vi "Arm Mode.vi"() -> ()   [LabVIEW 2015]
uses:
  Global Angle.vi
  Global Distance.vi
panel:
  in  "last 2":dbl
  in  "last":dbl
  out "delta1":dbl
  out "delta2":dbl
  out "delta3":dbl
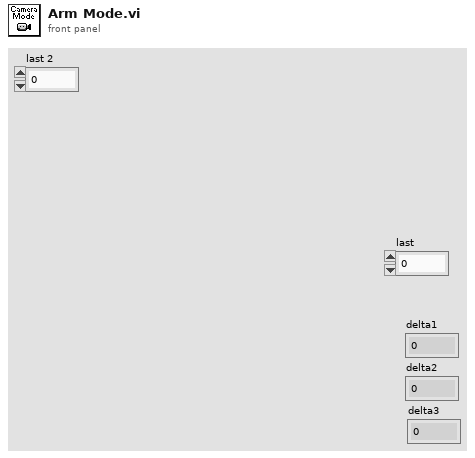
[diagram p1: front panel]
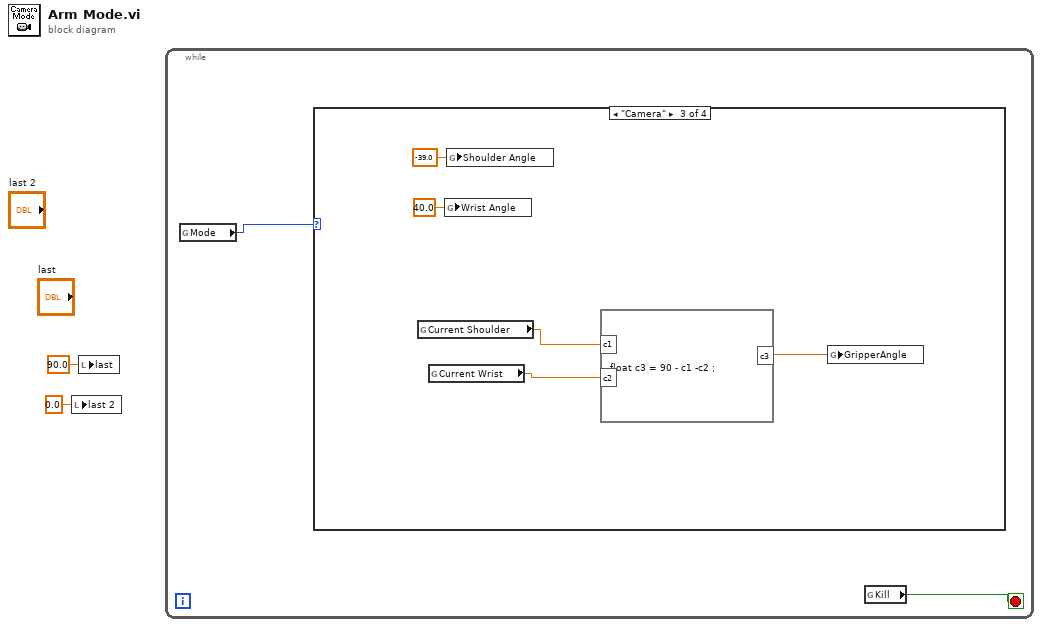
[diagram p0: block diagram]
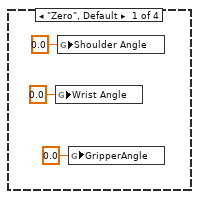
[diagram p2: hidden frame]
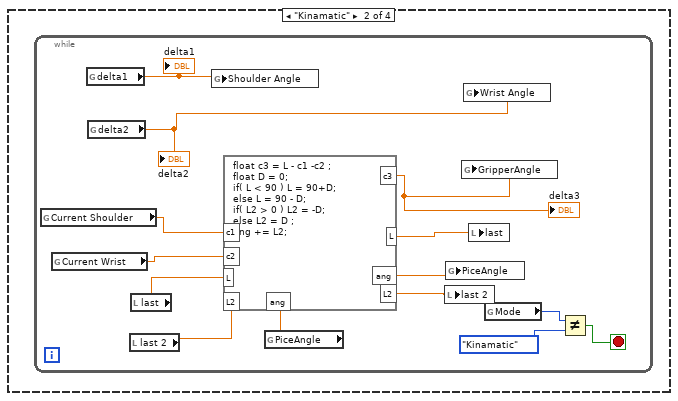
[diagram p3: hidden frame]
diagram:
  n1 = local write "last 2"(0.0 ("last 2")) -> ()
  n2 = local write "last"(90.0 ("last")) -> ()
  n3 = while {
    stop <- w3 stop-if-true
    n4 = global read "Global Angle.vi" "Mode"() -> (w4:enum16{"Normal", "Zero", "Kinamatic", "Camera"})
    n5 = case shown="\"Camera\"" w4 {
      frame "Zero", Default {
        n6 = global write "Global Angle.vi" "Wrist Angle"(0.0 ("Wrist Angle")) -> ()
        n7 = global write "Global Angle.vi" "Shoulder Angle"(0.0 ("Shoulder Angle")) -> ()
        n8 = global write "Global Angle.vi" "GripperAngle"(0.0 ("GripperAngle")) -> ()
      }
      frame "Kinamatic" {
        n9 = while {
          stop <- w16 stop-if-true
          n10 = global read "Global Angle.vi" "Current Shoulder"() -> (w19:dbl)
          n11 = global read "Global Angle.vi" "Current Wrist"() -> (w18:dbl)
          n12 = global read "Global Distance.vi" "delta1"() -> (w21:dbl)
          "delta1" <- w21
          n13 = global read "Global Distance.vi" "delta2"() -> (w20:dbl)
          "delta2" <- w20
          n14 = local read "last 2"() -> (w11:dbl)
          n15 = local read "last"() -> (w12:dbl)
          n16 = global write "Global Angle.vi" "Shoulder Angle"(w21) -> ()
          n17 = global read "Global Angle.vi" "PiceAngle"() -> (w10:dbl)
          n18 = formula code="float c3 = L - c1 -c2 ;\nfloat D = 0;\nif( L < 90 ) L = 90+D;\nelse L = 90 - D;\nif( L2 > 0 ) L2 = -D;\nelse L2 = D ;\nang += L2;"("c1"=w19, "c2"=w18, "L"=w12, "L2"=w11, "ang"=w10) -> ("c3"=w17:dbl, "L"=w13:dbl, "ang"=w9:dbl, "L2"=w8:dbl)
          "delta3" <- w17
          n19 = local write "last 2"(w8) -> ()
          n20 = global write "Global Angle.vi" "PiceAngle"(w9) -> ()
          n21 = global write "Global Angle.vi" "GripperAngle"(w17) -> ()
          n22 = global write "Global Angle.vi" "Wrist Angle"(w20) -> ()
          n23 = local write "last"(w13) -> ()
          n24 = global read "Global Angle.vi" "Mode"() -> (w14:enum16{"Normal", "Zero", "Kinamatic", "Camera"})
          n25 = Not Equal?(x=w14, y=enum16{"Zero", "Kinamatic", "Camera"}."Kinamatic") -> (x != y?=w16:bool)
        }
      }
      frame "Camera" {
        n26 = global read "Global Angle.vi" "Current Shoulder"() -> (w24:dbl)
        n27 = global read "Global Angle.vi" "Current Wrist"() -> (w23:dbl)
        n28 = global write "Global Angle.vi" "Wrist Angle"(40.0 ("Wrist Angle")) -> ()
        n29 = global write "Global Angle.vi" "Shoulder Angle"(-39.0 ("Shoulder Angle")) -> ()
        n30 = formula code="float c3 = 90 - c1 -c2 ;"("c1"=w24, "c2"=w23) -> ("c3"=w22:dbl)
        n31 = global write "Global Angle.vi" "GripperAngle"(w22) -> ()
      }
      frame "Normal" {
      }
    }
    n32 = global read "Global Angle.vi" "Kill"() -> (w3:bool)
  }
